vi "RTE-17_moose.vi"(2 "Send \nCommand":bool, 4 "Option Box":i32(listbox), 7 "Screen Control":bool=TRUE, 8 "Numerical\nSet Value":dbl format="%.2f") -> (1 "Numeric Return":dbl format="%.2f", 5 "Return Dialog":string)   [LabVIEW 2010]
doc: "This VI serves as a main interface panel between the user and any Neslab Chiller using binary serial communications (this package designed for the RTE-140 Refridgerated Bath/Circulator). All subVIs used in this VI were origionally contained within the same VI library. \nTo use this VI:\n- Highlight the desired function in the \"Option Box\"\n- If it is a \"Set\" function, enter the desired value in the \"Numerical Set Value,\" otherwise;\n- Select the \"Send Command\" boolean. \nRepeat steps as necessary.\nSelect the \"Close Screen\" boolean to quite the VI."
panel:
  out "error out 2":errorcluster
  in  "error in (no error)":errorcluster
  in  "COM Port":refnum<visa-resource-name>="COM12"
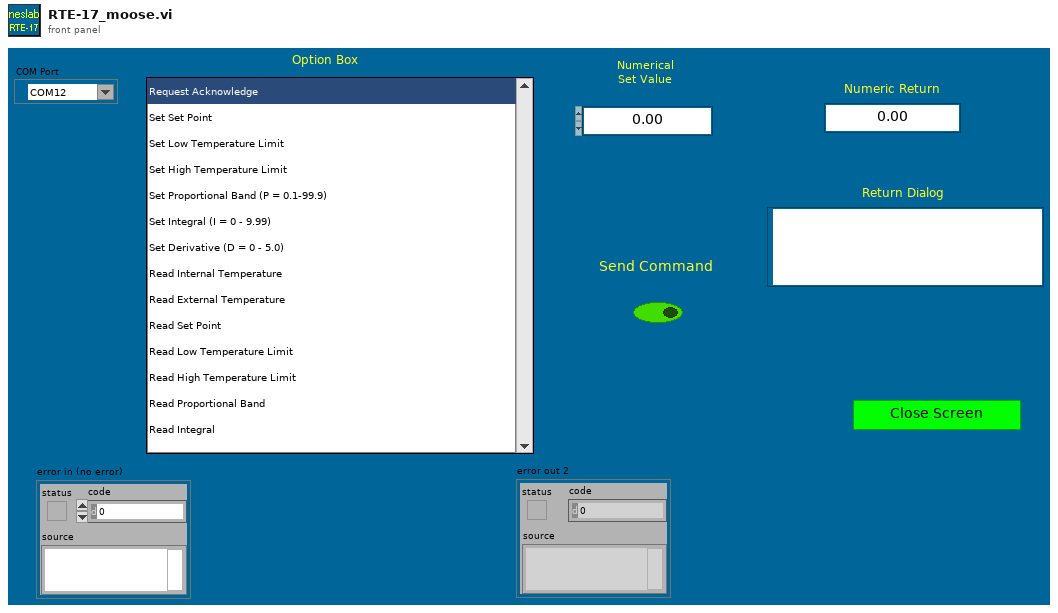
[diagram p1: front panel]
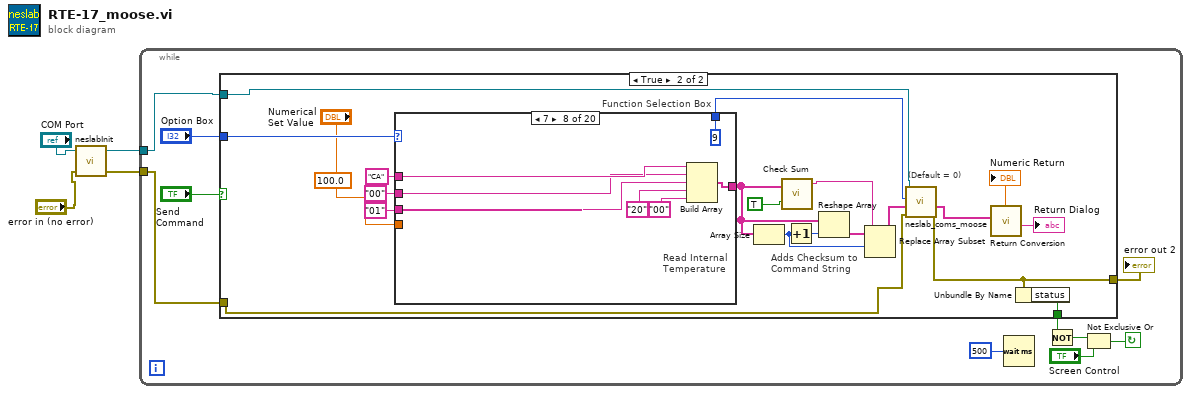
[diagram p0: block diagram]
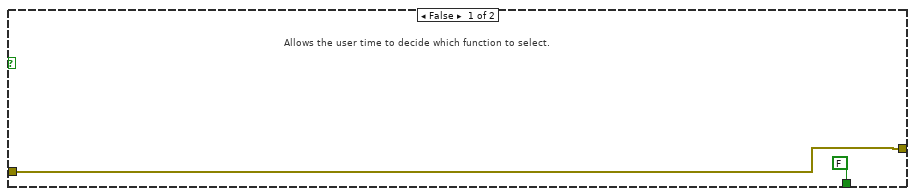
[diagram p2: hidden frame]
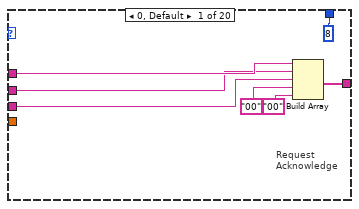
[diagram p3: hidden frame]
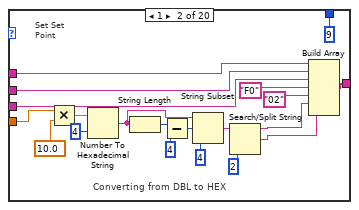
[diagram p4: hidden frame]
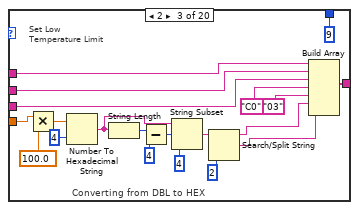
[diagram p5: hidden frame]
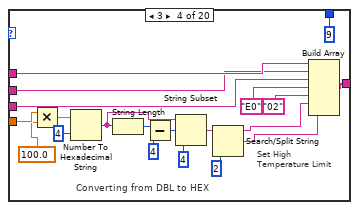
[diagram p6: hidden frame]
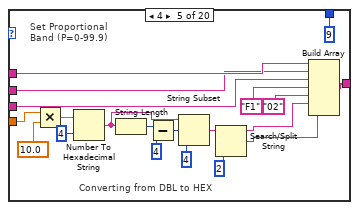
[diagram p7: hidden frame]
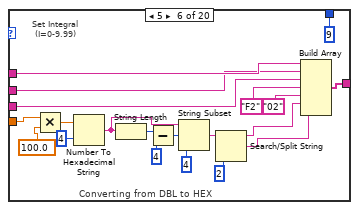
[diagram p8: hidden frame]
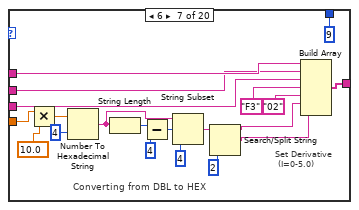
[diagram p9: hidden frame]
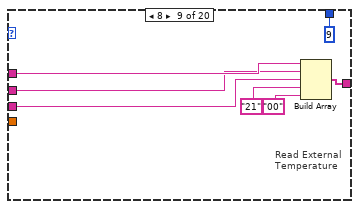
[diagram p10: hidden frame]
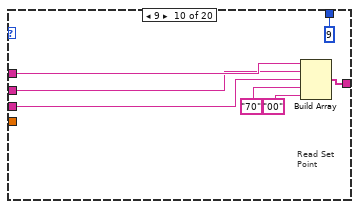
[diagram p11: hidden frame]
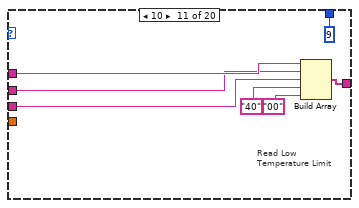
[diagram p12: hidden frame]
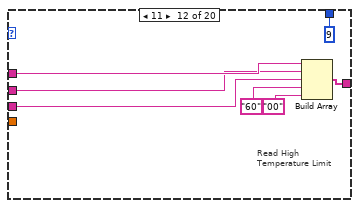
[diagram p13: hidden frame]
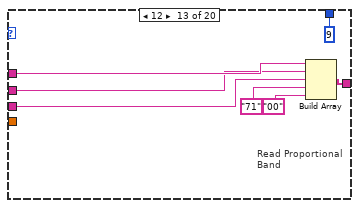
[diagram p14: hidden frame]
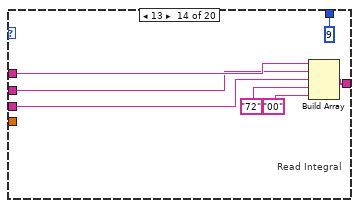
[diagram p15: hidden frame]
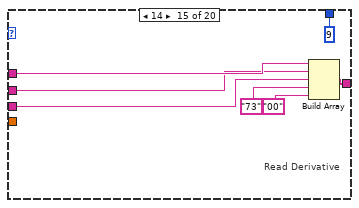
[diagram p16: hidden frame]
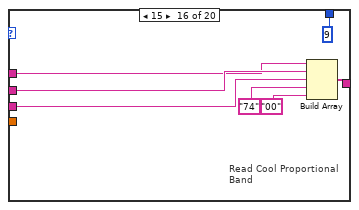
[diagram p17: hidden frame]
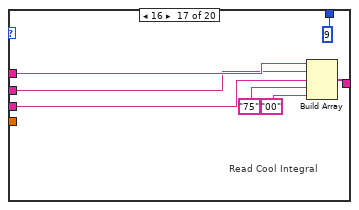
[diagram p18: hidden frame]
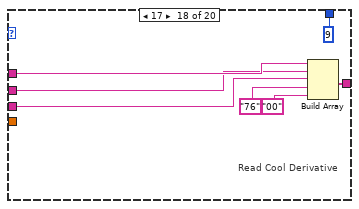
[diagram p19: hidden frame]
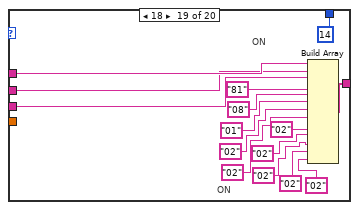
[diagram p20: hidden frame]
diagram:
  n1 = call "neslabInit.vi"("error in (no error)"="error in (no error)", "COM Port"="COM Port") -> ("error out"=w1:errorcluster, "COM Port Out"=w2:refnum<visa-resource-name>)  [unwired: 1 in, 1 out]
  n2 = while {
    tunnel: w2 -> [w7]
    tunnel: w1 -> [w6]
    stop <- w9 continue-if-true
    n3 = case shown="True" "Send \nCommand" {
      tunnel: "Option Box" -> [_ w25]
      tunnel: [w15 w19] -> w5
      tunnel: [FALSE w28] -> w8
      tunnel: w7 -> [_ w21]
      tunnel: w6 -> [w15 w20]
      frame False {
        # "Allows the user time to decide which function to select."
      }
      frame True {
        (unwired) 100.0 ("y")
        # "Adds Checksum to\nCommand String"
        # "Function Selection Box"
        # "(Default = 0)"
        n4 = case shown="7" w25 {
          tunnel: "CA" -> [w43 w63 w83 w103 w123 w143 w163 w170 w177 w184 w191 w198 w205 w212 w219 w220 w231 w237 w254 w269]
          tunnel: "00" -> [w42 w62 w82 w102 w122 w142 w162 w169 w176 w183 w190 w197 w204 w211 w218 w221 w227 w236 w253 w268]
          tunnel: "01" -> [w41 w61 w81 w101 w121 w141 w161 w168 w175 w182 w189 w196 w203 w210 w217 w223 w228 w235 w251 w266]
          tunnel: [w38 w58 w78 w98 w118 w138 w158 w165 w172 w179 w186 w193 w200 w207 w214 w222 w230 w238 w255 w270] -> w31
          tunnel: [u32 8 u32 9 u32 9 u32 9 u32 9 u32 9 u32 9 u32 9 u32 9 u32 9 u32 9 u32 9 u32 9 u32 9 u32 9 u32 9 u32 9 u32 9 u32 14 u32 14] -> w22
          tunnel: "Numerical\nSet Value" -> [_ w48 w68 w86 w108 w128 w146 _ _ _ _ _ _ _ _ _ _ _ _ _]
          frame 0, Default {
            # "Request\nAcknowledge"
            n5 = Build Array(w43, w42, w41, "00", "00") -> (w38:string[])
          }
          frame 1 {
            # "Converting from DBL to HEX"
            # "Set Set\nPoint"
            n6 = Multiply(x=w48, y=10.0) -> (x*y=w49:dbl)
            n7 = Number To Hexadecimal String(1:i16 4 ("width (-)"), 2:w49) -> (0:w44:string)
            n8 = String Length(string=w44) -> (length=w54:i32)
            n9 = Subtract(x=w54, y=4) -> (x-y=w53:i32)
            n10 = String Subset(string=w44, offset (0)=w53, length (rest)=4 ("length (rest)")) -> (substring=w50:string)
            n11 = Search/Split String(string=w50, offset (0)=2) -> (substring before match=w45:string, match + rest of string=w46:string)  [unwired: 1 in, 1 out]
            n12 = Build Array(w63, w62, w61, "F0", "02", w45, w46) -> (w58:string[])
          }
          frame 2 {
            # "Converting from DBL to HEX"
            # "Set Low \nTemperature Limit"
            n13 = Multiply(x=w68, y=100.0) -> (x*y=w69:dbl)
            n14 = Number To Hexadecimal String(1:i16 4 ("width (-)"), 2:w69) -> (0:w64:string)
            n15 = String Length(string=w64) -> (length=w74:i32)
            n16 = Subtract(x=w74, y=4) -> (x-y=w73:i32)
            n17 = String Subset(string=w64, offset (0)=w73, length (rest)=4 ("length (rest)")) -> (substring=w70:string)
            n18 = Search/Split String(string=w70, offset (0)=2) -> (substring before match=w66:string, match + rest of string=w65:string)  [unwired: 1 in, 1 out]
            n19 = Build Array(w83, w82, w81, "C0", "03", w66, w65) -> (w78:string[])
          }
          frame 3 {
            # "Converting from DBL to HEX"
            # "Set High\nTemperature Limit"
            n20 = Multiply(x=w86, y=100.0) -> (x*y=w89:dbl)
            n21 = Number To Hexadecimal String(1:i16 4 ("width (-)"), 2:w89) -> (0:w84:string)
            n22 = String Length(string=w84) -> (length=w94:i32)
            n23 = Subtract(x=w94, y=4) -> (x-y=w93:i32)
            n24 = String Subset(string=w84, offset (0)=w93, length (rest)=4 ("length (rest)")) -> (substring=w90:string)
            n25 = Search/Split String(string=w90, offset (0)=2) -> (substring before match=w88:string, match + rest of string=w87:string)  [unwired: 1 in, 1 out]
            n26 = Build Array(w103, w102, w101, "E0", "02", w88, w87) -> (w98:string[])
          }
          frame 4 {
            # "Converting from DBL to HEX"
            # "Set Proportional\nBand (P=0-99.9)"
            n27 = Multiply(x=w108, y=10.0 ("f")) -> (x*y=w109:dbl)
            n28 = Number To Hexadecimal String(1:i16 4 ("width (-)"), 2:w109) -> (0:w104:string)
            n29 = String Length(string=w104) -> (length=w114:i32)
            n30 = Subtract(x=w114, y=4) -> (x-y=w113:i32)
            n31 = String Subset(string=w104, offset (0)=w113, length (rest)=4 ("length (rest)")) -> (substring=w110:string)
            n32 = Search/Split String(string=w110, offset (0)=2) -> (substring before match=w106:string, match + rest of string=w105:string)  [unwired: 1 in, 1 out]
            n33 = Build Array(w123, w122, w121, "F1", "02", w106, w105) -> (w118:string[])
          }
          frame 5 {
            # "Converting from DBL to HEX"
            # "Set Integral\n (I=0-9.99)"
            n34 = Multiply(x=w128, y=100.0) -> (x*y=w129:dbl)
            n35 = Number To Hexadecimal String(1:i16 4 ("width (-)"), 2:w129) -> (0:w124:string)
            n36 = String Length(string=w124) -> (length=w134:i32)
            n37 = Subtract(x=w134, y=4) -> (x-y=w133:i32)
            n38 = String Subset(string=w124, offset (0)=w133, length (rest)=4 ("length (rest)")) -> (substring=w130:string)
            n39 = Search/Split String(string=w130, offset (0)=2) -> (substring before match=w127:string, match + rest of string=w126:string)  [unwired: 1 in, 1 out]
            n40 = Build Array(w143, w142, w141, "F2", "02", w127, w126) -> (w138:string[])
          }
          frame 6 {
            # "Converting from DBL to HEX"
            # "Set Derivative\n (I=0-5.0)"
            n41 = Multiply(x=w146, y=10.0 ("f")) -> (x*y=w149:dbl)
            n42 = Number To Hexadecimal String(1:i16 4 ("width (-)"), 2:w149) -> (0:w144:string)
            n43 = String Length(string=w144) -> (length=w154:i32)
            n44 = Subtract(x=w154, y=4) -> (x-y=w153:i32)
            n45 = String Subset(string=w144, offset (0)=w153, length (rest)=4 ("length (rest)")) -> (substring=w150:string)
            n46 = Search/Split String(string=w150, offset (0)=2) -> (substring before match=w148:string, match + rest of string=w147:string)  [unwired: 1 in, 1 out]
            n47 = Build Array(w163, w162, w161, "F3", "02", w148, w147) -> (w158:string[])
          }
          frame 7 {
            # "Read Internal\nTemperature"
            n48 = Build Array(w170, w169, w168, "20", "00") -> (w165:string[])
          }
          frame 8 {
            # "Read External\nTemperature"
            n49 = Build Array(w177, w176, w175, "21", "00") -> (w172:string[])
          }
          frame 9 {
            # "Read Set\nPoint"
            n50 = Build Array(w184, w183, w182, "70", "00") -> (w179:string[])
          }
          frame 10 {
            # "Read Low \nTemperature Limit"
            n51 = Build Array(w191, w190, w189, "40", "00") -> (w186:string[])
          }
          frame 11 {
            # "Read High\nTemperature Limit"
            n52 = Build Array(w198, w197, w196, "60", "00") -> (w193:string[])
          }
          frame 12 {
            # "Read Proportional\nBand"
            n53 = Build Array(w205, w204, w203, "71", "00") -> (w200:string[])
          }
          frame 13 {
            # "Read Integral"
            n54 = Build Array(w212, w211, w210, "72", "00") -> (w207:string[])
          }
          frame 14 {
            # "Read Derivative"
            n55 = Build Array(w219, w218, w217, "73", "00") -> (w214:string[])
          }
          frame 15 {
            # "Read Cool Proportional\nBand"
            n56 = Build Array(w220, w221, w223, "74", "00") -> (w222:string[])
          }
          frame 16 {
            # "Read Cool Integral"
            n57 = Build Array(w231, w227, w228, "75", "00") -> (w230:string[])
          }
          frame 17 {
            # "Read Cool Derivative"
            n58 = Build Array(w237, w236, w235, "76", "00") -> (w238:string[])
          }
          frame 18 {
            # "ON"
            # "ON"
            n59 = Build Array(w254, w253, w251, "81", "08", "01", "02", "02", "02", "02", "02", "02", "02") -> (w255:string[])
          }
          frame 19 {
            # "OFF"
            # "OFF"
            n60 = Build Array(w269, w268, w266, "81", "08", "00", "02", "02", "02", "02", "02", "02", "02") -> (w270:string[])
          }
        }
        n61 = Array Size(array=w31) -> (size(s)=w32:i32)
        n62 = call "Check Sum.VI"("Input String"=w31, "Append Checksum?"=TRUE) -> ("Checksum"=w26:string)  [unwired: 2 out]
        n63 = Increment(x=w32) -> (x+1=w33:i32)
        n64 = Reshape Array(w31, w33) -> (w34:string[])
        n65 = Replace Array Subset(array=w34, new element=w26, index=w32) -> (w23:string[])
        n66 = call "neslab_coms_moose.vi"("error in"=w20, "byte array\n(in)"=w23, "Bytes to Read"=w22, "COM Port IN"=w21) -> ("error out 2"=w19:errorcluster, "byte array\n(out)"=w18:string[])  [unwired: 2 in, 2 out]
        n67 = call "Return Conversion.VI"("Input Array"=w18) -> ("Numeric\nReading\nValue"=→"Numeric Return":dbl, "Reading String\nwith Descriptor"=→"Return Dialog":string)  [unwired: 7 in]
        n68 = Unbundle By Name(w19) -> ("status"=w28:bool)
      }
    }
    "error out 2" <- w5
    n69 = Wait (ms)(milliseconds to wait=u32 500 ("y")) -> ()  [unwired: 1 out]
    n70 = Not(x=w8) -> (.not. x?=w11:bool)
    n71 = Not Exclusive Or(1:"Screen Control", 2:w11) -> (0:w9:bool)
  }
